vi "Grava_Temp_TDC_u.vi"(2 "array 2D with data":u32[][](array[numeric]) format="%x", 3 "Folder path: Temp or TDC":path) -> (1 "quants arxius fets":i32)   [LabVIEW 2015, in "VIPM2.lvlib"]
doc: "Grava els Global Registers programats en arxius personalitzats per ChipID\n\" \\ChipID.txt \""
uses:
  VIPM2.lvlib
  <vilib>/Utility/file.llb/Write To Spreadsheet File (I64).vi
panel:
  # "Subrutina: grava les temperatures mesurades en arxius personalitzats per ChipID\n                   grava les TDC calibrations en arxius personalitzats per ChipID"
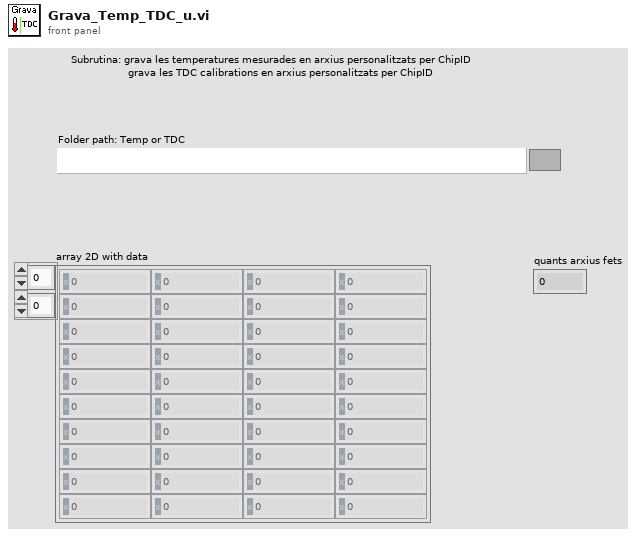
[diagram p1: front panel]
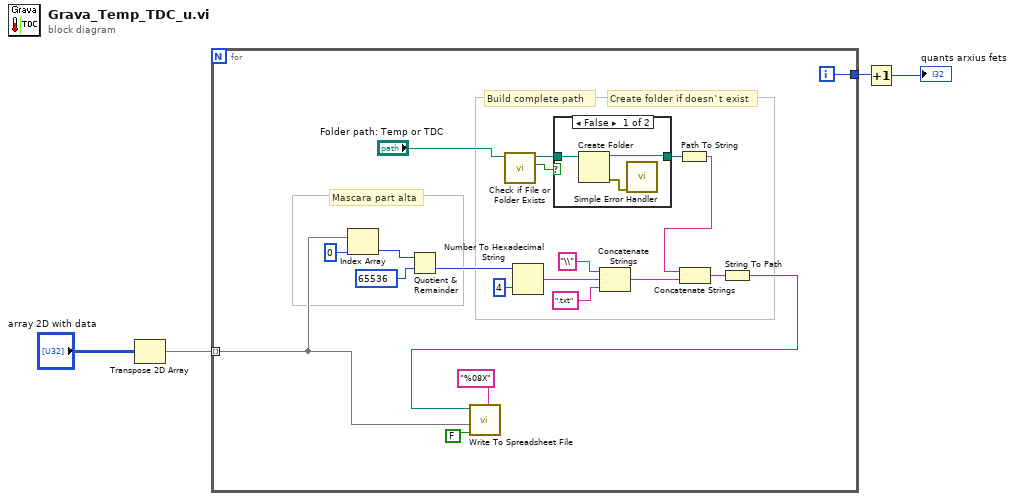
[diagram p0: block diagram]
diagram:
  n1 = Transpose 2D Array(2D array="array 2D with data") -> (transposed array=w2:u32[][])
  n2 = for {
    tunnel: [w13] -> w4
    tunnel: w2 -> [w5] mode=indexing
    i -> [w13]
    # "Create folder if doesn`t exist"
    # "Build complete path"
    # "Mascara part alta"
    n3 = Index Array(array=w5, index=0) -> (element=w6:u32)
    n4 = Quotient & Remainder(x=w6, y=u32 65536) -> (floor(x/y)=w23:u32)  [unwired: 1 out]
    n5 = call <vilib>:"Check if File or Folder Exists.vi"("path"="Folder path: Temp or TDC") -> ("file or folder exists?"=w12:bool, "dup path"=w11:path)  [unwired: 8 in, 1 out]
    n6 = Number To Hexadecimal String(1:i16 4 ("width (-)"), 2:w23) -> (0:w20:string)
    n7 = case shown="False" w12 {
      tunnel: w11 -> [w27 w28]
      tunnel: [w26 w28] -> w10
      frame False {
        n8 = Create Folder(path (use dialog)=w27) -> (created path=w26:path, error out=w25:errorcluster)  [unwired: 2 in, 1 out]
        n9 = call <vilib>:"Simple Error Handler.vi"("error in (no error)"=w25) -> ()  [unwired: 4 in, 5 out]
      }
      frame True {
      }
    }
    n10 = Concatenate Strings("\\" ("string"), w20, ".txt" ("string")) -> (w16:string)
    n11 = Path To String(path=w10) -> (string=w8:string)
    n12 = Concatenate Strings(w8, w16) -> (w15:string)
    n13 = String To Path(string=w15) -> (path=w14:path)
    n14 = call-poly <vilib>:"Write To Spreadsheet File.vi"("format (%d)"="%08X", "append to file? (new file:F)"=FALSE, "1D data"=w5, "file path (dialog if empty)"=w14) -> ()  [unwired: 4 in, 1 out]
  }
  n15 = Increment(x=w4) -> (x+1=→"quants arxius fets":i32)
